vi "Cleanup.vi"(8 "error in (no error)":errorcluster, 11 "Manager in":refnum<class "Manager.lvclass">) -> (0 "error out":errorcluster, 1 "Events":dbl, 2 "Wait Done":dbl)   [LabVIEW 2020, in "OOPanel.lvlib" / "Manager.lvclass"]
uses:
  Manager.lvclass
  Manager.lvclass/Manager.ctl
  Panel/Close Reason.ctl
  Panel/Panel.lvclass
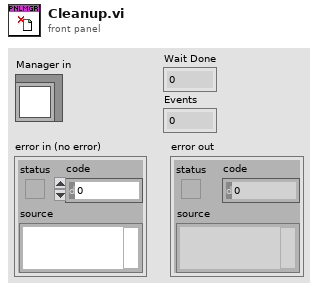
[diagram p1: front panel]
types:
  T1 = typedef "OOPanel.lvlib/Manager.lvclass/Ref Data.ctl" = cluster{"SubPanel Map":T2, "Panels":refnum<class "Panel.lvclass">[]}
  T2 = typedef "OOPanel.lvlib/Manager.lvclass/SubPanel Map.ctl" = cluster{"SubPanels":refnum<vi>[], "Panels":refnum<class "Panel.lvclass">[]}
  T3 = typedef "OOPanel.lvlib/Panel.lvclass/Close Reason.ctl" = enum16{"Shutdown", "Close"}
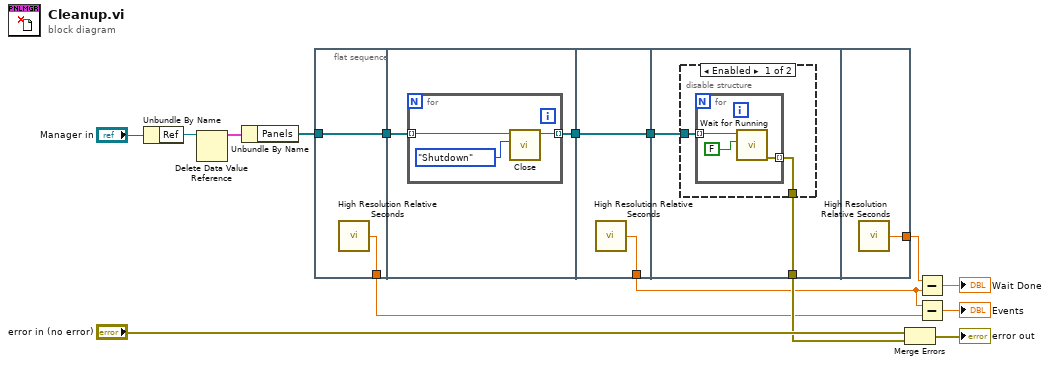
[diagram p0: block diagram]
diagram:
  n1 = Unbundle By Name("Manager in") -> ("Ref"=w13:refnum<data-value>)
  n2 = Delete Data Value Reference(data value reference=w13) -> (data value=w12:T1)  [unwired: 1 in, 1 out]
  n3 = Unbundle By Name(w12) -> ("Panels"=w10:refnum<class "Panel.lvclass">[])
  n4 = flat-sequence {
    tunnel: w10 -> [w17]
    tunnel: [w17] -> w6
    tunnel: [w16] -> w3
    tunnel: [w18] -> w7
    tunnel: w6 -> [w19]
    tunnel: [w24] -> w8
    tunnel: w7 -> [w24]
    tunnel: [w23] -> w4
    tunnel: [w26] -> w9
    tunnel: w8 -> [w25]
    tunnel: [w32] -> w5
    frame #0 {
      n5 = call <vilib>:"High Resolution Relative Seconds.vi"() -> ("relative seconds"=w16:dbl)
    }
    frame #1 {
      n6 = for {
        tunnel: w19 -> [w22] mode=indexing
        tunnel: [w20] -> w18 mode=indexing
        n7 = call "Close.vi"("Reason"=Close_Reason."Shutdown", "Panel in"=w22) -> ("Panel out"=w20:refnum<class "Panel.lvclass">)  [unwired: 8 in, 1 out]
      }
    }
    frame #2 {
      n8 = call <vilib>:"High Resolution Relative Seconds.vi"() -> ("relative seconds"=w23:dbl)
    }
    frame #3 {
      n9 = disable-structure shown="Enabled" {
        disable-tunnel: [w28 _] -> w26
        disable-tunnel: w25 -> [w27 _]
        frame Enabled {
          n10 = for {
            tunnel: [w30] -> w28 mode=indexing
            tunnel: w27 -> [w29] mode=indexing
            n11 = call "Wait for Running.vi"("Running"=FALSE, "Panel in"=w29) -> ("error out"=w30:errorcluster)  [unwired: 8 in, 1 out]
          }
        }
        frame Disabled {
        }
      }
    }
    frame #4 {
      n12 = call <vilib>:"High Resolution Relative Seconds.vi"() -> ("relative seconds"=w32:dbl)
    }
  }
  n13 = Merge Errors("error in (no error)", w9) -> (→"error out":errorcluster)
  n14 = Subtract(x=w5, y=w4) -> (x-y=→"Wait Done":dbl)
  n15 = Subtract(x=w4, y=w3) -> (x-y=→"Events":dbl)
